vi "_24_Sample_qsns_10[4].vi"() -> ()   [LabVIEW 2020]
panel:
  out "min index(es)":i32
  out "min value":i32
  out "max index(es)":i32
  out "max value":i32
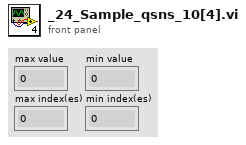
[diagram p1: front panel]
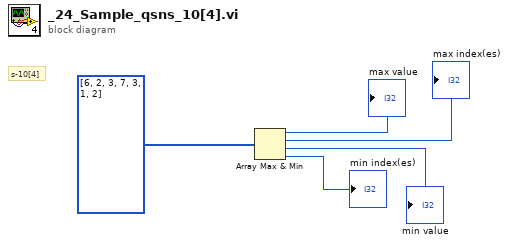
[diagram p0: block diagram]
diagram:
  # "s-10[4]"
  n1 = Array Max & Min(array=i32[] [6, 2, 3, 7, 3, 1, 2] ("Array 2")) -> (max value=→"max value":i32, max index (indices)=→"max index(es)":i32, min value=→"min value":i32, min index (indices)=→"min index(es)":i32)
